vi "MainFormLauncher.vi"() -> ()   [LabVIEW 2024]
uses:
  MFActor/MFActor/MFActor.lvclass
panel:
  out "String":string
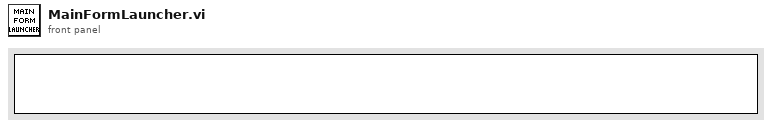
[diagram p1: front panel]
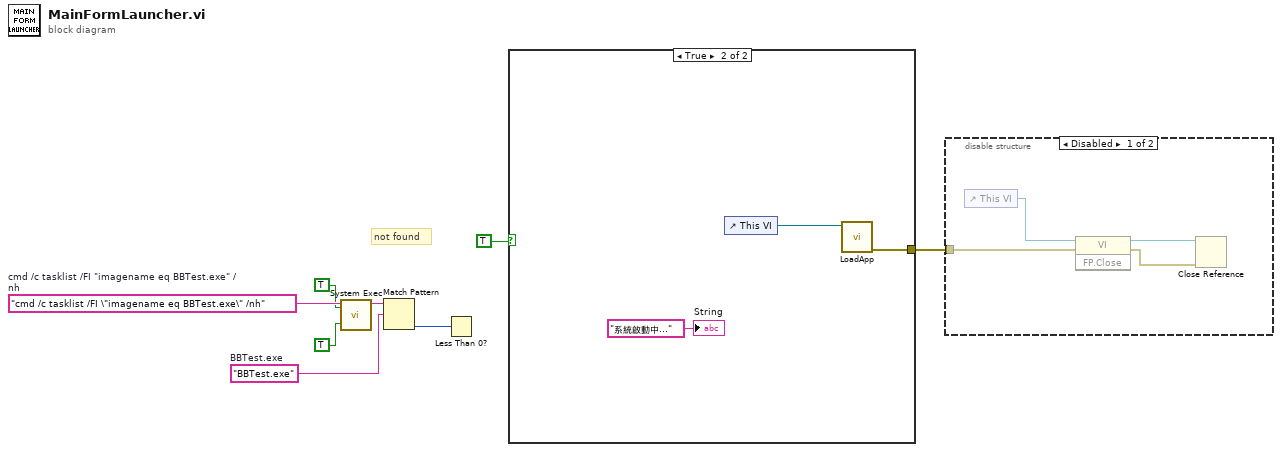
[diagram p0: block diagram]
diagram:
  w4 = "BBTest.exe"  # BBTest.exe
  w8 = "cmd /c tasklist /FI \"imagename eq BBTest.exe\" /nh"  # cmd /c tasklist /FI "imagename eq BBTest.exe" /nh
  # "not found"
  n1 = call <vilib>:"System Exec.vi"("run minimized? (F)"=TRUE, "wait until completion? (T)"=TRUE, "command line"=w8) -> ("standard output"=w5:string)  [unwired: 5 in, 3 out]
  n2 = Match Pattern(string=w5, regular expression=w4) -> (offset past match=w3:i32)  [unwired: 1 in, 3 out]
  n3 = Less Than 0?(x=w3) -> ()  [unwired: 1 out]
  n4 = case shown="True" TRUE {
    tunnel: [_ w10] -> w2
    frame False {
    }
    frame True {
      n5 = control-ref of="This VI"() -> (w9:refnum<vi>)
      n6 = call "LoadApp.vi"("Launcher"=w9) -> ("error out"=w10:errorcluster)  [unwired: 10 in]
      "String" <- "系統啟動中..." ("String")
    }
  }
  n7 = disable-structure shown="Disabled" {
    disable-tunnel: w2 -> [w12 _]
    frame Disabled {
      n8 = control-ref of="This VI"() -> (w13:refnum<vi>)
      n9 = invoke class="VI" method="FP.Close"(reference=w13, error in=w12) -> (reference out=w14:refnum<vi>, error out=w15:errorcluster)  [unwired: 1 in, 1 out]
      n10 = Close Reference(reference=w14, error in (no error)=w15) -> ()  [unwired: 1 out]
    }
    frame Enabled {
    }
  }
